vi "Receiver.vi"() -> ()   [LabVIEW 2020]
uses:
  DataType.ctl
  Receiver/Receiver.lvclass
panel:
  out "Error Out":errorcluster
  out "Received?":bool
  out "Value":T1 {"Tank 5" scale=0.0..255.0; "Tank 4" scale=0.0..255.0; "Tank 3" scale=0.0..255.0; "Tank 2" scale=0.0..255.0; "Tank" scale=0.0..255.0}
  in  "Stop":bool
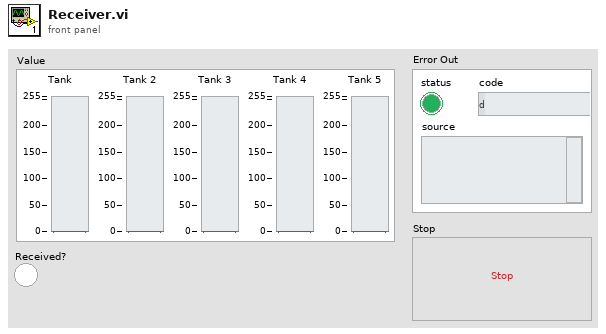
[diagram p1: front panel]
types:
  T1 = typedef "DataType.ctl" = cluster{"Tank":u8, "Tank 2":u8, "Tank 3":u8, "Tank 4":u8, "Tank 5":u8}
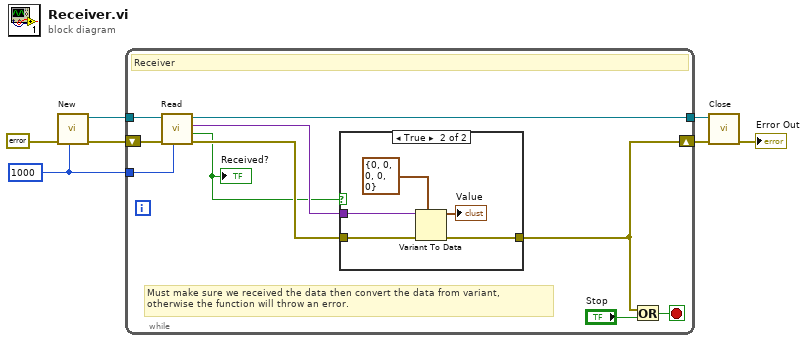
[diagram p0: block diagram]
diagram:
  w3 = 1000 ("Timeout ms (25000)")
  n1 = call "New.vi"("Timeout ms (25000)"=w3, "Error In"=errorcluster {"status"=FALSE, "code"=0, "source"=""}) -> ("Error Out"=w7:errorcluster, "Receiver Ref."=w6:refnum<class "Receiver.lvclass">)  [unwired: 8 in]
  n2 = while {
    shift-right: [w9] -> w5
    shift-left: w7 -> [w17]
    tunnel: w6 -> [w16]
    tunnel: [w15] -> w4
    tunnel: w3 -> [w14]
    stop <- w12 stop-if-true
    # "Must make sure we received the data then convert the data from variant,\notherwise the function will throw an error."
    # "Receiver"
    n3 = call "Read.vi"("Timeout ms (1000)"=w14, "Error In"=w17, "Receiver Ref."=w16) -> ("Error Out"=w11:errorcluster, "Received?"=w8:bool, "Value"=w10:variant, "Receiver Ref."=w15:refnum<class "Receiver.lvclass">)  [unwired: 5 in]
    "Received?" <- w8
    n4 = case shown="True" w8 {
      tunnel: w11 -> [w18 w23]
      tunnel: w10 -> [_ w22]
      tunnel: [w18 w21] -> w9
      frame False {
      }
      frame True {
        n5 = Variant To Data(error in=w23, type=T1 {"Tank"=0, "Tank 2"=0, "Tank 3"=0, "Tank 4"=0, "Tank 5"=0} ("Data"), Variant=w22) -> (data=→"Value":T1, error out=w21:errorcluster)
      }
    }
    n6 = Or(x=w9, y="Stop") -> (x .or. y?=w12:bool)
  }
  n7 = call "Close.vi"("Error In"=w5, "Receiver Ref."=w4) -> ("Error Out"=→"Error Out":errorcluster)  [unwired: 9 in]
